vi "Update Start Position.vi"(8 "error in (no error)":errorcluster, 10 "Position":T1, 11 "Team Config Panel in":refnum<class "Team Config Panel.lvclass">) -> (0 "error out":errorcluster, 3 "Team Config Panel out":refnum<class "Team Config Panel.lvclass">)   [LabVIEW 2020, in "SB App.lvlib" / "Team Config Panel.lvclass"]
uses:
  Team Config Panel.lvclass
  SquareBattle/Position.ctl
  Team Config Panel.lvclass/Team Config Panel.ctl
  SquareBattle/SquareBattle.lvlib
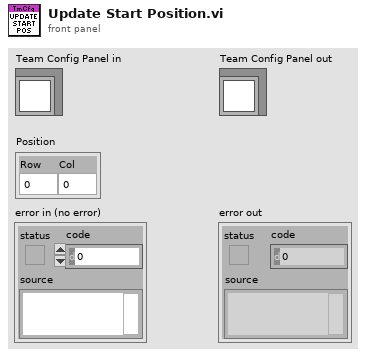
[diagram p1: front panel]
types:
  T1 = typedef "SquareBattle.lvlib/Position.ctl" = cluster{"Row":i32, "Col":i32}
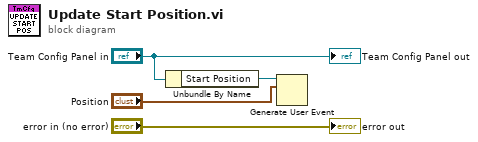
[diagram p0: block diagram]
diagram:
  n1 = Unbundle By Name("Team Config Panel in") -> ("Start Position"=w2:refnum<user-event>)
  n2 = Generate User Event(user event=w2, event data cluster="Position") -> ()  [unwired: 2 in, 2 out]
  "error out" <- "error in (no error)"
  "Team Config Panel out" <- "Team Config Panel in"
